vi "softIOC.vi"(8 "error in (no error)":errorcluster caption="错误输入（无错误）", 11 "路径":path) -> (0 "error out":errorcluster, 3 "IOC started":bool)   [LabVIEW 2013]
uses:
  <vilib>/Utility/error.llb/DialogType.ctl
  <userlib>/caLab/lib/caLabIoc.dll
panel:
  in  "Minimize IOC":bool=TRUE caption="minimize IOC (T)"
  out "Command Line":string
  out "Result":string
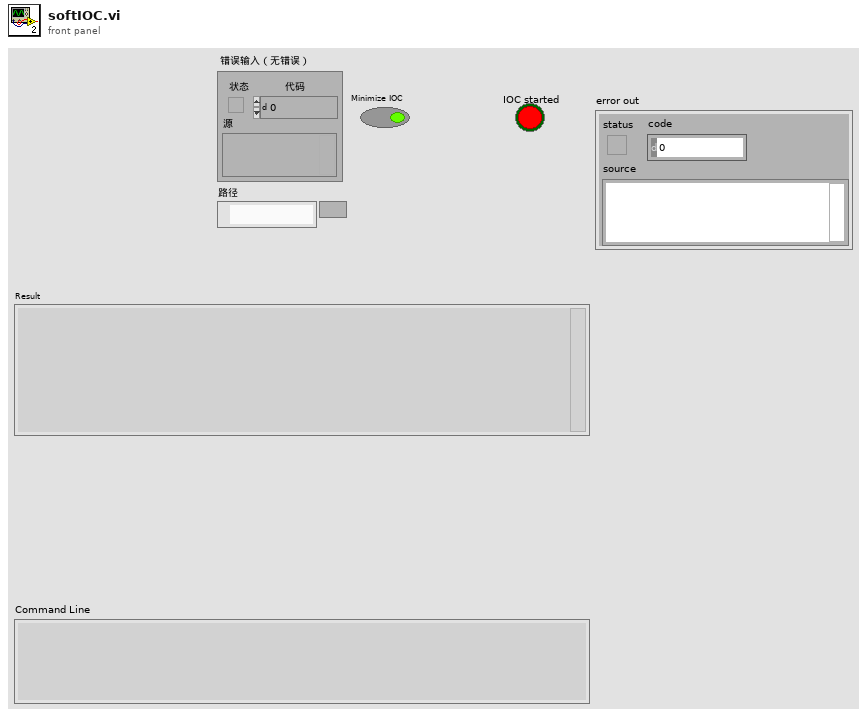
[diagram p1: front panel]
types:
  T1 = typedef "DialogType.ctl" = u16
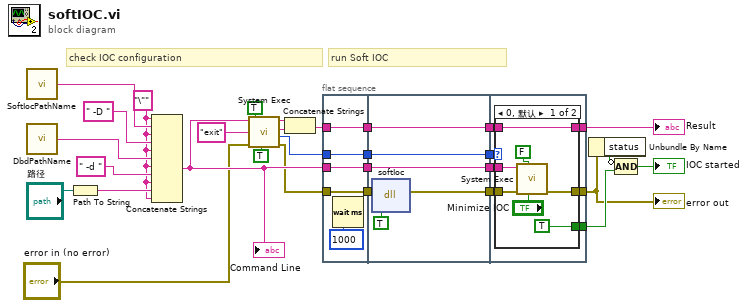
[diagram p0: block diagram]
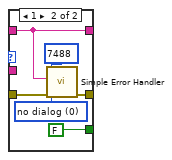
[diagram p2: hidden frame]
diagram:
  w3 = "\""
  # "run Soft IOC"
  # "check IOC configuration"
  n1 = call <userlib>:"SoftIocPathName.vi"() -> ("pathName"=w8:string)  [unwired: 1 out]
  n2 = call <userlib>:"DbdPathName.vi"() -> ("pathName"=w6:string)  [unwired: 1 out]
  n3 = Path To String(path="路径") -> (string=w4:string)
  n4 = Concatenate Strings(w3, w8, w3, " -D " ("string"), w3, w6, w3, " -d " ("string"), w3, w4, w3) -> (w15:string)
  "Command Line" <- w15
  n5 = call <vilib>:"System Exec.vi"("run minimized? (F)"=TRUE, "wait until completion? (T)"=TRUE, "error in (no error)"="error in (no error)", "standard input"="exit", "command line"=w15) -> ("error out"=w13:errorcluster, "return code"=w19:i32, "standard error"=w20:string, "standard output"=w21:string)  [unwired: 1 in, 2 out]
  n6 = Concatenate Strings(w21, w20) -> (w12:string)
  n7 = flat-sequence {
    tunnel: w13 -> [w32]
    tunnel: w15 -> [w33]
    tunnel: w19 -> [w34]
    tunnel: w12 -> [w35]
    tunnel: [w35] -> w30
    tunnel: [w34] -> w29
    tunnel: [w33] -> w28
    tunnel: [w32] -> w27
    tunnel: [w41] -> w26
    tunnel: [w40] -> w25
    tunnel: [w39] -> w24
    tunnel: [w37] -> w23
    tunnel: w30 -> [w41]
    tunnel: w29 -> [w40]
    tunnel: w28 -> [w39]
    tunnel: w27 -> [w38]
    tunnel: [w48] -> w22
    tunnel: [w46] -> w10
    tunnel: w26 -> [w47]
    tunnel: w25 -> [w45]
    tunnel: w24 -> [w44]
    tunnel: w23 -> [w43]
    tunnel: [w42] -> w11
    frame #0 {
      n8 = Wait (ms)(milliseconds to wait=u32 1000) -> ()  [unwired: 1 out]
    }
    frame #1 {
      n9 = dll-call lib="D:/Program Files (x86)/National Instruments/LabVIEW 2013/user.lib/caLab/lib/caLabIoc.dll" fn="softIoc"(error in=w38, "forceOneIOC"=TRUE) -> (error out=w37:errorcluster)  [unwired: 2 in, 3 out]
    }
    frame #2 {
      n10 = case shown="0, 默认" w45 {
        tunnel: w44 -> [w53 _]
        tunnel: [TRUE FALSE] -> w48
        tunnel: w47 -> [w49 w56]
        tunnel: [w51 w58] -> w46
        tunnel: w43 -> [w50 w57]
        tunnel: [w49 w56] -> w42
        frame 0, Default {
          n11 = call <vilib>:"System Exec.vi"("run minimized? (F)"="Minimize IOC", "wait until completion? (T)"=FALSE, "error in (no error)"=w50, "command line"=w53) -> ("error out"=w51:errorcluster)  [unwired: 2 in, 5 out]
        }
        frame 1 {
          w60 = T1 0 items=["no dialog", "OK message", "continue or stop message", "OK message + warnings", "continue/stop + warnings"] ("type of dialog (OK msg:1)")
          n12 = call <vilib>:"Simple Error Handler.vi"("error code (no error:0)"=7488, "error source (\" \")"=w56, "type of dialog (OK msg:1)"=w60, "error in (no error)"=w57) -> ("error out"=w58:errorcluster)  [unwired: 5 out]
        }
      }
    }
  }
  n13 = Unbundle By Name(w10) -> ("status"=w14:bool)
  n14 = Compound Arithmetic op=AND(invert w14, w22) -> (→"IOC started":bool)
  "error out" <- w10
  "Result" <- w11
